vi "svx_Polar_Align_All.vi"(4 "Previous Selector Visible?":bool, 6 "Current Container bounds":cluster{"Width":u32, "Height":u32}, 7 "Display State In":T1={"Property Name"=[], "Container bounds"={"Width"=550, "Height"=250}, "Scale range"={"Maximum"=1.0, "Increment"=1.0}, "PointIdx"=0, "Marker list"=[], "Color settings"={"Arrow color"=16860, "Magnitude major grid"=13816530, "Magnitude minor grid"=16777216, "Phase grid"=13816530, "Phase scale marker text"=0}, "Magnitude scale name"="Magnitude", "Magnitude scale format string"="%#.2e", "MagnitudeScale:Visible"=TRUE, "MagnitudeScaleLabel:Visible"=TRUE, "PhaseScale:Visible"=TRUE, "Marker:Visible"=TRUE, "Cursor:Visible"=FALSE, "CursorName:Visible"=TRUE, "Autoscale"=TRUE, "Marker color"=16860, "Line color"=16711680, "Cursor color"=16711680, "Magnitude scale marker color"=0, "Plot.Line Style"=0, "Plot.Line Width"=0, "Plot.Point Style"=0, "Cursor.Line Style"=0, "Cursor.Line Width"=0, "Cursor.Point Style"=0, "Cursor.Style"=4, "Marker.Point Style"=2, "Point/fill color"=16711680, "Background color"=16777225, "Cursor name"="", "Cursor Release"=refnum, "Scale Range Change"=refnum, "data size(s)"=[], "Selectors:Visible"=TRUE, "Selector:ring Strings"={"Selector:Custom Strings"=FALSE, "Selector:Row Strings []"=[], "Selector:Column Strings []"=[], "User:Row Strings []"=[], "User:Column Strings []"=[]}, "Lock Cursor Info Position"=FALSE, "CursLoc"={"magnitude"=0.0, "phase"=0.0, "time/rev/RPM"=0.0}, "Plot Area:Position"={"Left"=0, "Top"=0}, "Plot Area:Size"={"Width"=0, "Height"=0}, "Marker.Style"=0, "Indication Arcs"=[], "Arc.Selector"=0, "customized marker"=[], "tree Width"=0, " Parents Tags"=[], "Children Tags"=[], "open?"=[], "index"=[{"row index"=0, "column index"=0}], "Label"="", "custom strings changed"=FALSE, "Owning VI"=refnum, "Legend BG color"=16777225, "Legend font color"=0, "column Width"=203, "attribute"=variant}, 8 "z scale graph Refnum":refnum<vi>, 9 "Plot Legend Refnum":refnum<vi>, 10 "Polar Plot ref in":refnum<vi>, 11 "Container Refnum":refnum<vi>) -> (0 "z scale graph Refnum out":refnum<vi>, 1 "Plot Legend Refnum out":refnum<vi>, 2 "Polar Plot ref out":refnum<vi>, 3 "Container Refnum out":refnum<vi>, 5 "Display State out":T1={"Property Name"=[], "Container bounds"={"Width"=550, "Height"=250}, "Scale range"={"Maximum"=1.0, "Increment"=1.0}, "PointIdx"=0, "Marker list"=[], "Color settings"={"Arrow color"=16860, "Magnitude major grid"=13816530, "Magnitude minor grid"=16777216, "Phase grid"=13816530, "Phase scale marker text"=0}, "Magnitude scale name"="Magnitude", "Magnitude scale format string"="%#.2e", "MagnitudeScale:Visible"=TRUE, "MagnitudeScaleLabel:Visible"=TRUE, "PhaseScale:Visible"=TRUE, "Marker:Visible"=TRUE, "Cursor:Visible"=FALSE, "CursorName:Visible"=TRUE, "Autoscale"=TRUE, "Marker color"=16860, "Line color"=16711680, "Cursor color"=16711680, "Magnitude scale marker color"=0, "Plot.Line Style"=0, "Plot.Line Width"=0, "Plot.Point Style"=0, "Cursor.Line Style"=0, "Cursor.Line Width"=0, "Cursor.Point Style"=0, "Cursor.Style"=4, "Marker.Point Style"=2, "Point/fill color"=16711680, "Background color"=16777225, "Cursor name"="", "Cursor Release"=refnum, "Scale Range Change"=refnum, "data size(s)"=[], "Selectors:Visible"=TRUE, "Selector:ring Strings"={"Selector:Custom Strings"=FALSE, "Selector:Row Strings []"=[], "Selector:Column Strings []"=[], "User:Row Strings []"=[], "User:Column Strings []"=[]}, "Lock Cursor Info Position"=FALSE, "CursLoc"={"magnitude"=0.0, "phase"=0.0, "time/rev/RPM"=0.0}, "Plot Area:Position"={"Left"=0, "Top"=0}, "Plot Area:Size"={"Width"=0, "Height"=0}, "Marker.Style"=0, "Indication Arcs"=[], "Arc.Selector"=0, "customized marker"=[], "tree Width"=0, " Parents Tags"=[], "Children Tags"=[], "open?"=[], "index"=[{"row index"=0, "column index"=0}], "Label"="", "custom strings changed"=FALSE, "Owning VI"=refnum, "Legend BG color"=16777225, "Legend font color"=0, "column Width"=203, "attribute"=variant} caption="State")   [LabVIEW 2017, in "SVX Polar Plot.xctl"]
uses:
  <vilib>/addons/_XControls/Polar Plot/SVX Polar Plot.xctl
  <vilib>/addons/_XControls/Polar Plot/subVIs/svx_Polar_Plot_Internal_State.ctl
  <vilib>/addons/_XControls/Polar Plot/subVIs/svx_Polar_Indication_Arcs.ctl
  <vilib>/addons/_XControls/Polar Plot/subVIs/svx_Polar_Customized_Markers.ctl
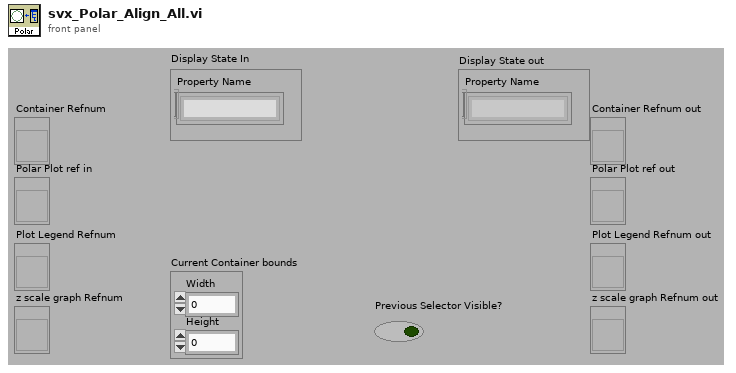
[diagram p1: front panel]
types:
  T1 = typedef "SVX Polar Plot.xctl/svx_Polar_Plot_Internal_State.ctl" = cluster{"Property Name":string[], "Container bounds":cluster{"Width":u32, "Height":u32}, "Scale range":cluster{"Maximum":dbl, "Increment":dbl}, "PointIdx":i32, "Marker list":cluster{"Name":string, "Color":u32, "Style":u8, "Point Style":u8, "Name Visible":bool, "Allow Drag":bool, "Annotation Mode":u32, "Plot":i32, "Index":i32, "Position":cluster{"X":dbl, "Y":dbl}, "X Scale":u32, "Y Scale":u32, "Show Arrow":bool, "Lock Name":bool, "Plot Area":i32, "Label Offset":cluster{"X":dbl, "Y":dbl}}[], "Color settings":cluster{"Arrow color":u32, "Magnitude major grid":u32, "Magnitude minor grid":u32, "Phase grid":u32, "Phase scale marker text":u32}, "Magnitude scale name":string, "Magnitude scale format string":string, "MagnitudeScale:Visible":bool, "MagnitudeScaleLabel:Visible":bool, "PhaseScale:Visible":bool, "Marker:Visible":bool, "Cursor:Visible":bool, "CursorName:Visible":bool, "Autoscale":bool, "Marker color":u32, "Line color":u32, "Cursor color":u32, "Magnitude scale marker color":u32, "Plot.Line Style":i32, "Plot.Line Width":i32, "Plot.Point Style":i32, "Cursor.Line Style":i32, "Cursor.Line Width":i32, "Cursor.Point Style":i32, "Cursor.Style":i32, "Marker.Point Style":i32, "Point/fill color":u32, "Background color":u32, "Cursor name":string, "Cursor Release":refnum<user-event>, "Scale Range Change":refnum<user-event>, "data size(s)":i32[], "Selectors:Visible":bool, "Selector:ring Strings":cluster{"Selector:Custom Strings":bool, "Selector:Row Strings []":string[], "Selector:Column Strings []":string[], "User:Row Strings []":string[], "User:Column Strings []":string[]}, "Lock Cursor Info Position":bool, "CursLoc":cluster{"magnitude":dbl, "phase":dbl, "time/rev/RPM":dbl}, "Plot Area:Position":cluster{"Left":i32, "Top":i32}, "Plot Area:Size":cluster{"Width":u32, "Height":u32}, "Marker.Style":i32, "Indication Arcs":T2, "Arc.Selector":u16, "customized marker":T3, "tree Width":u32, " Parents Tags":string[], "Children Tags":string[], "open?":bool[], "index":cluster{"row index":i32, "column index":i32}[], "Label":string, "custom strings changed":bool, "Owning VI":refnum<vi>, "Legend BG color":u32, "Legend font color":u32, "column Width":u32, "attribute":variant}
  T2 = typedef "SVX Polar Plot.xctl/svx_Polar_Indication_Arcs.ctl" = cluster{"Name":string, "Start radius":dbl, "End radius":dbl, "Line Style":i32, "Line Width":i32, "Border color":u32, "Fill color":u32, "Start angle":i16, "End angle":i16, "Visible":bool}[]
  T3 = typedef "SVX Polar Plot.xctl/svx_Polar_Customized_Markers.ctl" = cluster{"Name":string, "Color":u32, "Style":u8, "Point Style":u8, "Name Visible":bool, "Allow Drag":bool, "Annotation Mode":u32, "Plot":i32, "Index":i32, "Position":cluster{"Magnitude":dbl, "Phase":dbl}, "X Scale":u32, "Y Scale":u32, "Show Arrow":bool, "Lock Name":bool, "Plot Area":i32, "Label Offset":cluster{"Magnitude":dbl, "Phase":dbl}}[]
  T4 = typedef "LVRectTypeDef.ctl" = cluster{"Left":i16, "Top":i16, "Right":i16, "Bottom":i16}
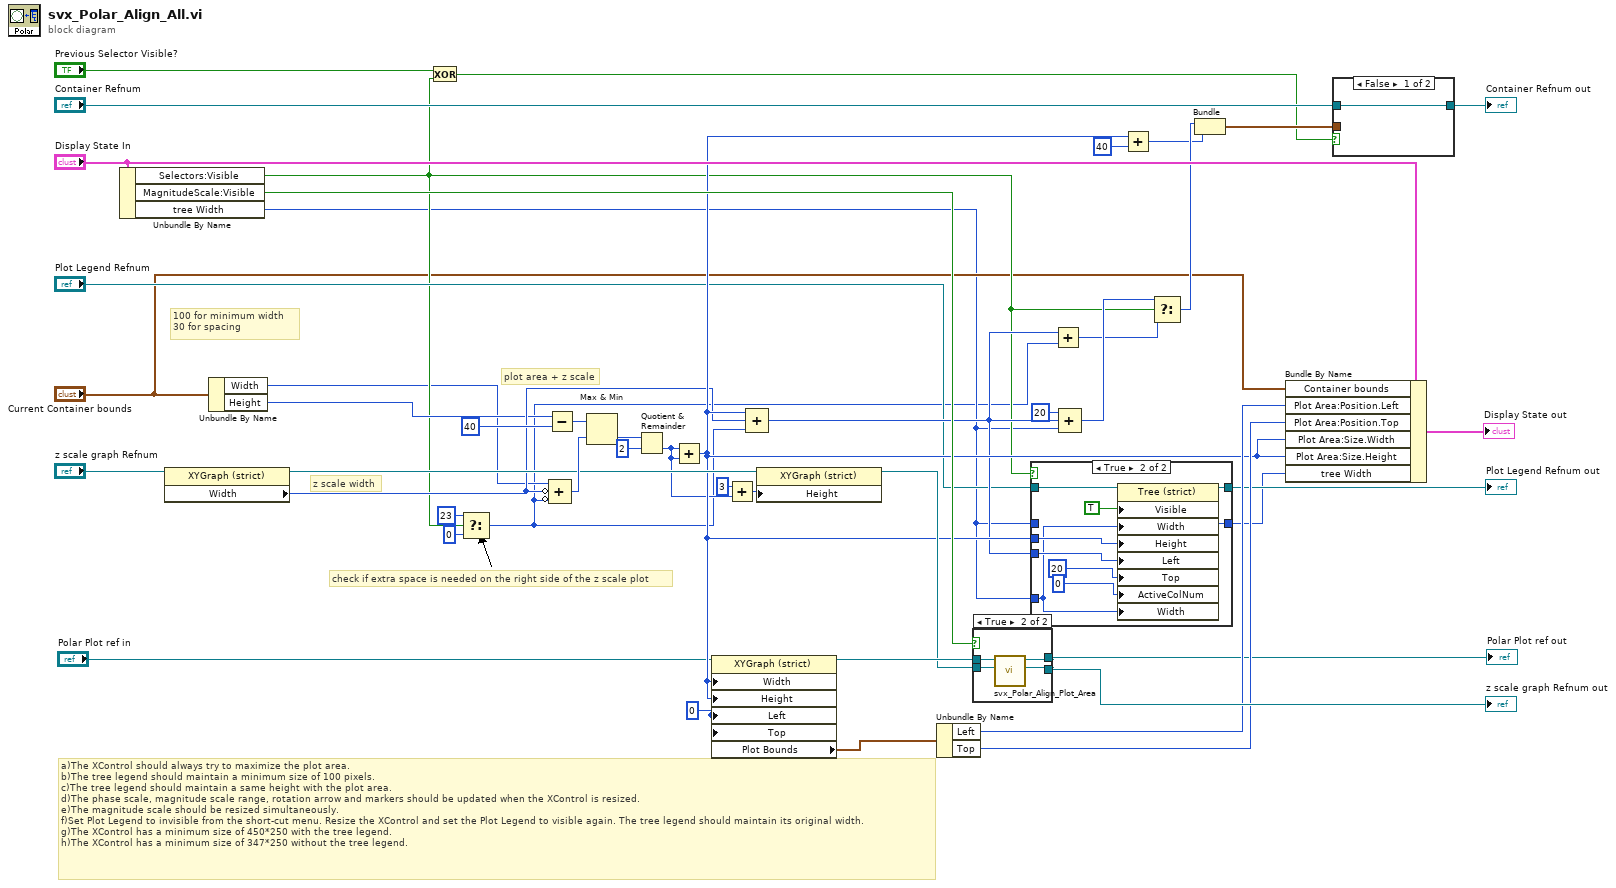
[diagram p0: block diagram]
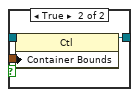
[diagram p2: hidden frame]
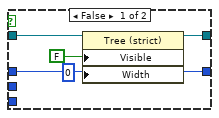
[diagram p3: hidden frame]
diagram:
  w41 = 0 ("Position:Left")
  # "check if extra space is needed on the right side of the z scale plot"
  # "a)The XControl should always try to maximize the plot area.\nb)The tree legend should maintain a minimum size of 100 pixels.\nc)The tree legend should maintain a same height with the plot area.\nd)The phase scale, magnitude scale range, rotation arrow and markers should be updated when the XControl is resized.\ne)The magnitude scale should be resized simultaneously.\nf)Set Plot Legend to invisible from the short-cut menu. Resize the XControl and set the Plot Legend to visible again. The tree legend should maintain its original width.\ng)The XControl has a minimum size of 450*250 with the tree legend.\nh)The XControl has a minimum size of 347*250 without the tree legend."
  # "z scale width"
  # "plot area + z scale"
  # "100 for minimum width\n30 for spacing"
  n1 = Unbundle By Name("Display State In") -> ("Selectors:Visible"=w9:bool, "MagnitudeScale:Visible"=w35:bool, "tree Width"=w4:u32)
  n2 = property class="XYGraph (strict)"(reference="z scale graph Refnum") -> (reference out=w40:refnum<vi>, "Width"=w23:u32)  [unwired: 1 in, 1 out]
  n3 = Unbundle By Name("Current Container bounds") -> ("Width"=w5:u32, "Height"=w18:u32)
  n4 = Exclusive Or(1:w9, 2:"Previous Selector Visible?") -> (0:w7:bool)
  n5 = Select(t=u32 23 ("value"), s=w9, f=u32 0) -> (s? t:f=w3:u32)
  n6 = Subtract(x=w18, y=i16 40) -> (x-y=w45:u32)
  n7 = Compound Arithmetic op=ADD(w5, invert w23, invert w3) -> (w44:u32)
  n8 = Max & Min(x=w45, y=w44) -> (min(x,y)=w42:u32)  [unwired: 1 out]
  n9 = Quotient & Remainder(x=w42, y=i16 2) -> (floor(x/y)=w24:u32)  [unwired: 1 out]
  n10 = Add(x=w24, y=w24) -> (x+y=w27:u32)
  n11 = property on="Property Node" class="XYGraph (strict)"(reference="Polar Plot ref in", "Width"=w27, "Height"=w27, "Left"=w41, "Top"=w41) -> (reference out=w37:refnum<vi>, "Plot Bounds"=w30:T4)  [unwired: 1 in, 1 out]
  n12 = Add(x=i16 3, y=w24) -> (x+y=w38:u32)
  n13 = Compound Arithmetic op=ADD(w27, w23, w3) -> (w20:u32)
  n14 = property class="XYGraph (strict)"(reference=w40, "Height"=w38) -> (reference out=w36:refnum<vi>)  [unwired: 1 in, 1 out]
  n15 = Unbundle By Name(w30) -> ("Left"=w29:i16, "Top"=w28:i16)
  n16 = case shown="True" w35 {
    tunnel: w37 -> [w49 w53]
    tunnel: w36 -> [w48 w52]
    tunnel: [w48 w51] -> w32
    tunnel: [w49 w50] -> w1
    frame False {
    }
    frame True {
      n17 = call <vilib>:"svx_Polar_Align_Plot_Area.vi"("z scale graph ref in"=w52, "Polar Plot ref in"=w53) -> ("z scale graph ref out"=w51:refnum<vi>, "Polar Plot ref out"=w50:refnum<vi>)  [unwired: 8 in]
    }
  }
  "z scale graph Refnum out" <- w32
  "Polar Plot ref out" <- w1
  n18 = case shown="True" w9 {
    tunnel: w27 -> [_ w66]
    tunnel: [w57 w65] -> w25
    tunnel: w20 -> [_ w64]
    tunnel: "Plot Legend Refnum" -> [w58 w63]
    tunnel: w4 -> [_ w59]
    tunnel: [w55 w59] -> w14
    tunnel: w4 -> [w55 _]
    frame False {
      n19 = property class="Tree (strict)"(reference=w58, "Visible"=FALSE, "Width"=u32 0 ("Size:Width")) -> (reference out=w57:refnum<vi>)  [unwired: 1 in, 1 out]
    }
    frame True {
      n20 = property class="Tree (strict)"(reference=w63, "Visible"=TRUE, "Width"=w59, "Height"=w66, "Left"=w64, "Top"=20 ("Position:Left"), "ActiveColNum"=0 ("Active Cell:Active Column Number"), "Width"=w59) -> (reference out=w65:refnum<vi>)  [unwired: 1 in, 1 out]
    }
  }
  "Plot Legend Refnum out" <- w25
  n21 = Add(x=w20, y=w3) -> (x+y=w19:u32)
  n22 = Compound Arithmetic op=ADD(20 ("value"), w20, w4) -> (w22:u32)
  n23 = Add(x=w27, y=40) -> (x+y=w16:u32)
  n24 = Select(t=w22, s=w9, f=w19) -> (s? t:f=w17:u32)
  n25 = Bundle(w17, w16) -> (w12:cluster{u32, u32})  [unwired: 1 in]
  n26 = Bundle By Name(cluster="Display State In", "Container bounds"="Current Container bounds", "Plot Area:Position.Left"=w29, "Plot Area:Position.Top"=w28, "Plot Area:Size.Width"=w27, "Plot Area:Size.Height"=w27, "tree Width"=w14) -> (→"Display State out":T1)
  n27 = case shown="False" w7 {
    tunnel: [w67 w70] -> w33
    tunnel: w12 -> [_ w69]
    tunnel: "Container Refnum" -> [w67 w68]
    frame False {
    }
    frame True {
      n28 = property class="Ctl"(reference=w68, "Container Bounds"=w69) -> (reference out=w70:refnum<vi>)  [unwired: 1 in, 1 out]
    }
  }
  "Container Refnum out" <- w33
